vi "Gauss2.vi"(0 "x":dbl[](array[numeric]), 1 "a5":dbl, 2 "a6":dbl, 5 "a1":dbl, 7 "a2":dbl, 9 "a3":dbl, 11 "a4":dbl) -> (4 "x+y":dbl[](array[numeric]))   [LabVIEW 2015]
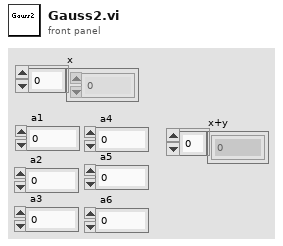
[diagram p1: front panel]
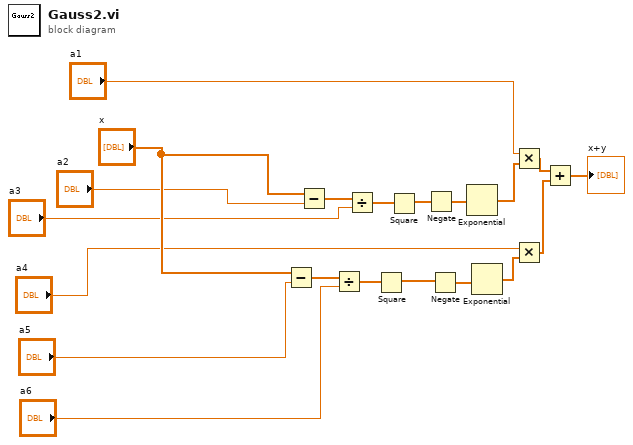
[diagram p0: block diagram]
diagram:
  n1 = Subtract(x="x", y="a5") -> (x-y=w17:dbl[])
  n2 = Subtract(x="x", y="a2") -> (x-y=w20:dbl[])
  n3 = Divide(x=w17, y="a6") -> (x/y=w16:dbl[])
  n4 = Divide(x=w20, y="a3") -> (x/y=w19:dbl[])
  n5 = Square(x=w16) -> (x^2=w12:dbl[])
  n6 = Square(x=w19) -> (x^2=w10:dbl[])
  n7 = Negate(x=w10) -> (-x=w9:dbl[])
  n8 = Negate(x=w12) -> (-x=w11:dbl[])
  n9 = Exponential(1:w9) -> (0:w18:dbl[])
  n10 = Exponential(1:w11) -> (0:w15:dbl[])
  n11 = Multiply(x="a1", y=w18) -> (x*y=w14:dbl[])
  n12 = Multiply(x="a4", y=w15) -> (x*y=w13:dbl[])
  n13 = Add(x=w14, y=w13) -> (x+y=→"x+y":dbl[])
